vi "AVI to Images.vi"() -> ()   [LabVIEW 2021]
uses:
  <vilib>/vision/Avi.llb/IMAQ AVI2 Codec Path.ctl
panel:
  out "error out":errorcluster
  out "AVI File Path":path=path "C:/Users/user/Documents/gest.avi/Image 2023_01_09_093516,831.avi"
  out "Image Out":T1(plugin-control)
  in  "Stop Button":bool
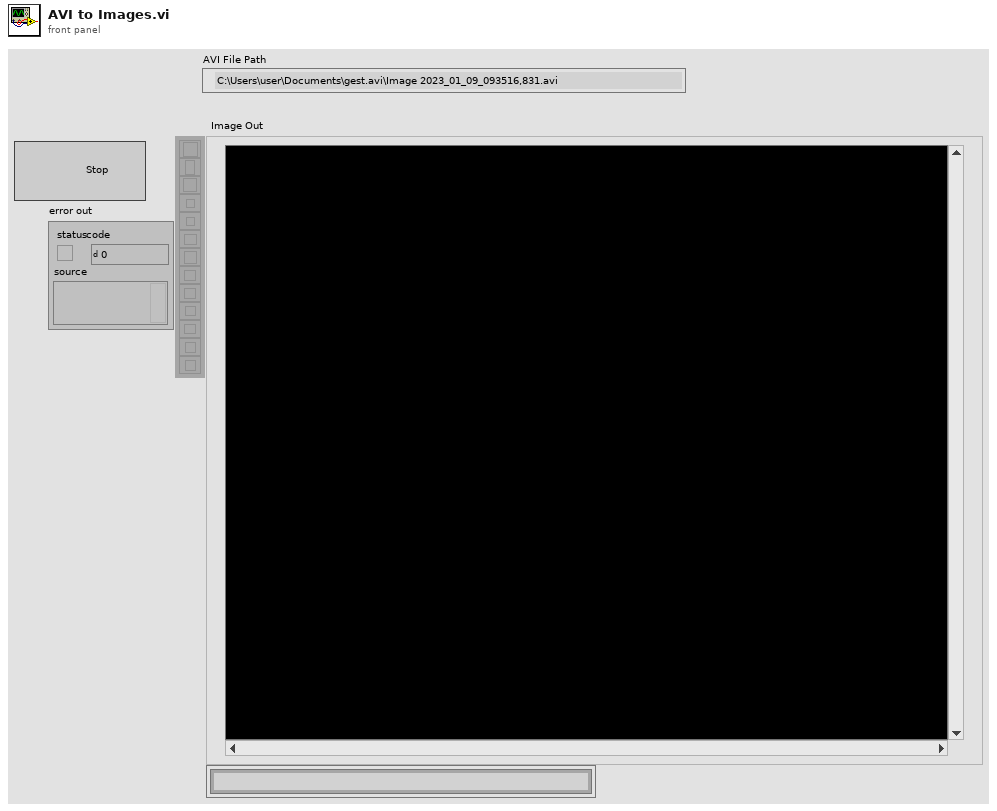
[diagram p1: front panel]
types:
  T1 = typedef "IMAQ Image.ctl" = refnum<image>
  T2 = typedef "IMAQ AVI2 Codec Path.ctl" = u32
  T3 = typedef "Image Type" = u32
  T4 = typedef "IMAQ AVI2 Refnum.ctl" = refnum<k20>
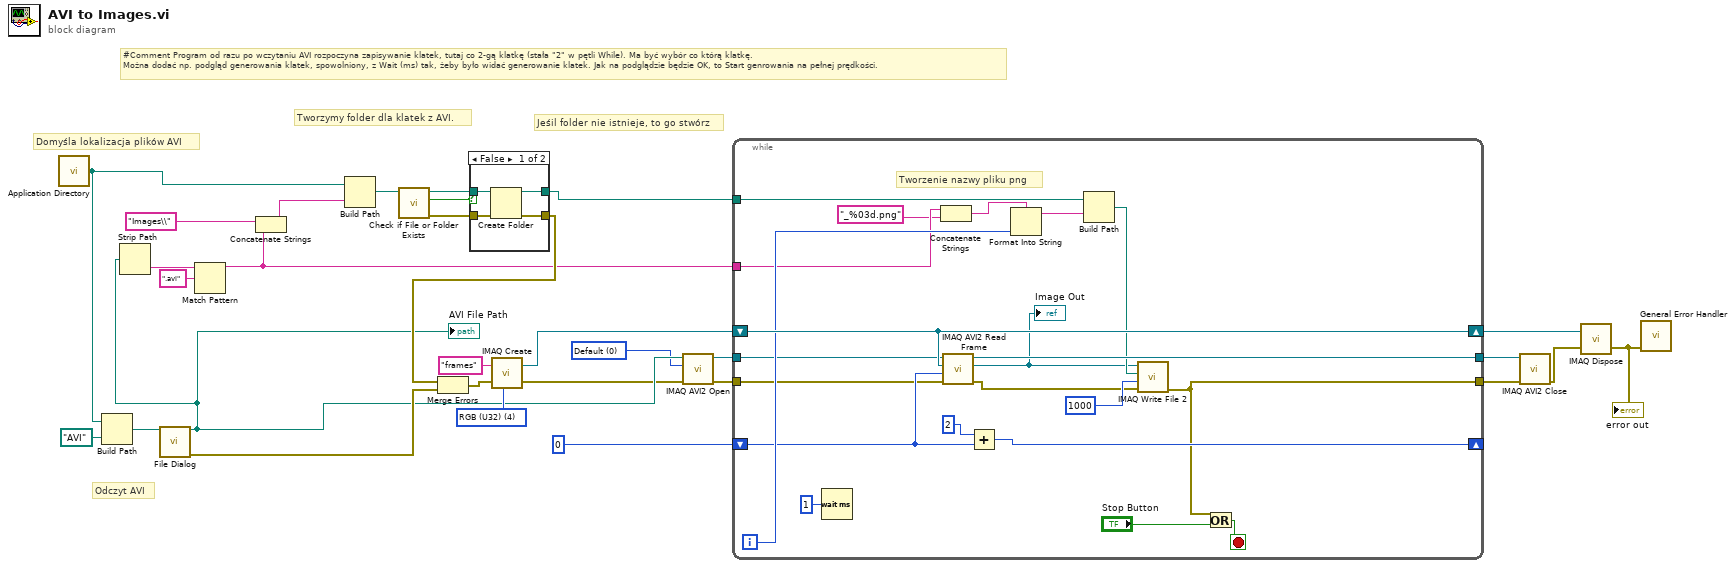
[diagram p0: block diagram]
diagram:
  w3 = T2 0 items=["Default", "System", "Built in Vision"] ("Codec Source")
  w29 = T3 4 items=["Grayscale (U8)", "Grayscale (I16)", "Grayscale (SGL)", "Complex (CSG)", "RGB (U32)", "HSL (U32)", "RGB (U64)", "Grayscale (U16)"] ("Image Type")
  # "Jeśil folder nie istnieje, to go stwórz"
  # "Tworzymy folder dla klatek z AVI."
  # "Domyśla lokalizacja plików AVI"
  # "Odczyt AVI"
  # "#Comment Program od razu po wczytaniu AVI rozpoczyna zapisywanie klatek, tutaj co 2-gą klatkę (stała \"2\" w pętli While). Ma być wybór co którą klatkę. \nMożna dodać np. podgląd generowania klatek, spowolniony, z Wait (ms) tak, żeby było widać generowanie klatek. Jak na podglądzie będzie OK, to Start genrowania na pełnej prędkości."
  n1 = call <vilib>:"Application Directory.vi"() -> ("Application Directory"=w15:path)
  n2 = Build Path(base path=w15, name or relative path=path "AVI") -> (appended path=w13:path)
  n3 = call "File Dialog"("start path"=w13) -> ("selected path"=w10:path, "error out"=w11:errorcluster)  [unwired: 11 in, 2 out]
  "AVI File Path" <- w10
  n4 = Strip Path(path=w10) -> (name=w7:string)  [unwired: 1 out]
  n5 = Match Pattern(string=w7, regular expression=".avi") -> (before substring=w5:string)  [unwired: 1 in, 3 out]
  n6 = Concatenate Strings("Images\\", w5) -> (w8:string)
  n7 = Build Path(base path=w15, name or relative path=w8) -> (appended path=w21:path)
  n8 = call <vilib>:"Check if File or Folder Exists.vi"("path"=w21) -> ("error out"=w19:errorcluster, "file or folder exists?"=w20:bool, "dup path"=w18:path)  [unwired: 8 in]
  n9 = case shown="False" w20 {
    tunnel: w19 -> [w34 w35]
    tunnel: w18 -> [w33 w36]
    tunnel: [w32 w36] -> w17
    tunnel: [w31 w35] -> w16
    frame False {
      n10 = Create Folder(path (use dialog)=w33, error in=w34) -> (created path=w32:path, error out=w31:errorcluster)  [unwired: 1 in, 1 out]
    }
    frame True {
    }
  }
  n11 = Merge Errors(w16, w11) -> (w12:errorcluster)
  n12 = call "IMAQ Create"("Image Name"="frames", "Image Type"=w29, "error in (no error)"=w12) -> ("New Image"=w27:T1, "error out"=w4:errorcluster)  [unwired: 2 in]
  n13 = call "IMAQ AVI2 Open"("error in (no error)"=w4, "Codec Source"=w3, "AVI File Path"=w10) -> ("error out"=w2:errorcluster, "AVI Refnum"=w1:T4)  [unwired: 7 in]
  n14 = while {
    shift-right: [w56] -> _
    shift-left: 0 -> [w44]
    tunnel: [w45] -> w25
    tunnel: [w55] -> w26
    tunnel: w17 -> [w43]
    tunnel: w5 -> [w42]
    shift-right: [w54] -> w23
    shift-left: w27 -> [w54]
    tunnel: w2 -> [w38]
    tunnel: w1 -> [w37]
    i -> [w50]
    stop <- w53 stop-if-true
    # "Tworzenie nazwy pliku png"
    n15 = Wait (ms)(milliseconds to wait=u32 1) -> ()  [unwired: 1 out]
    n16 = Concatenate Strings(w42, "_%03d.png" ("format string")) -> (w40:string)
    n17 = call "IMAQ AVI2 Read Frame"("error in (no error)"=w38, "Frame Number"=w44, "Image"=w54, "AVI Refnum"=w37) -> ("error out"=w46:errorcluster, "Image Out"=w39:T1, "AVI Refnum (duplicate)"=w55:T4)  [unwired: 5 in]
    "Image Out" <- w39
    n18 = Add(x=2, y=w44) -> (x+y=w56:i32)
    n19 = Format Into String(format string=w40, w50) -> (resulting string=w49:string)  [unwired: 2 in, 1 out]
    n20 = Build Path(base path=w43, name or relative path=w49) -> (appended path=w48:path)
    n21 = call-poly "IMAQ Write File 2"("error in (no error)"=w46, "Image Quality"=u32 1000, "File Path"=w48, "Image"=w39) -> ("error out"=w45:errorcluster)  [unwired: 6 in, 1 out]
    n22 = Or(x=w45, y="Stop Button") -> (x .or. y?=w53:bool)
  }
  n23 = call "IMAQ AVI2 Close"("error in (no error)"=w25, "AVI Refnum"=w26) -> ("error out"=w24:errorcluster)  [unwired: 9 in]
  n24 = call "IMAQ Dispose"("Image"=w23, "error in (no error)"=w24) -> ("error out"=w22:errorcluster)  [unwired: 4 in]
  "error out" <- w22
  n25 = call <vilib>:"General Error Handler.vi"("error in (no error)"=w22) -> ()  [unwired: 10 in, 5 out]
